vi "Medidor_File3.vi"() -> ()   [LabVIEW 2020]
uses:
  <vilib>/numeric/Random Number (Range) DBL.vi
panel:
  out "Potência C":dbl[](array[numeric])
  out "Corrente C":dbl[](array[numeric])
  out "Tensão C":dbl[](array[numeric])
  out "Potência Ativa C":dbl[](graph)
  out "Potência B":dbl[](array[numeric])
  out "Corrente B":dbl[](array[numeric])
  out "Tensão B":dbl[](array[numeric])
  out "Potência Ativa B":dbl[](graph)
  out "Potência Ativa":dbl[](array[numeric])
  out "Corrente A":dbl[](array[numeric])
  out "Tensão A":dbl[](array[numeric])
  out "Fator de potência":dbl
  in  "Limite inferior fp":dbl
  in  "Limite Superior FP":dbl=100.0
  out "Potência Ativa A":dbl[](graph)
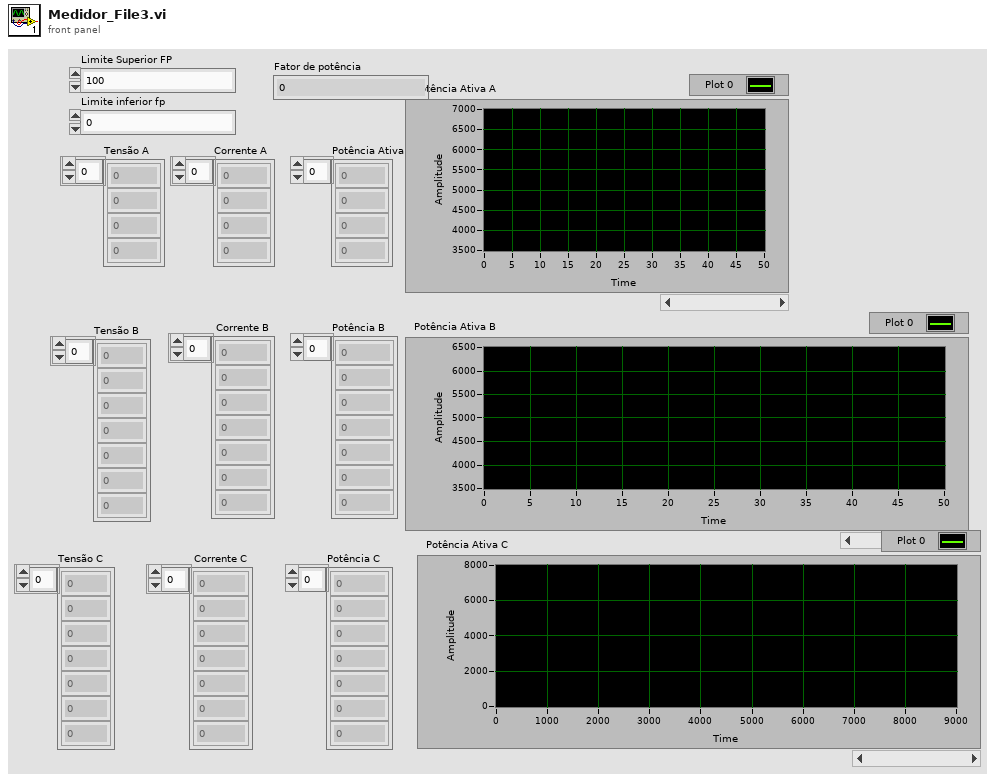
[diagram p1: front panel]
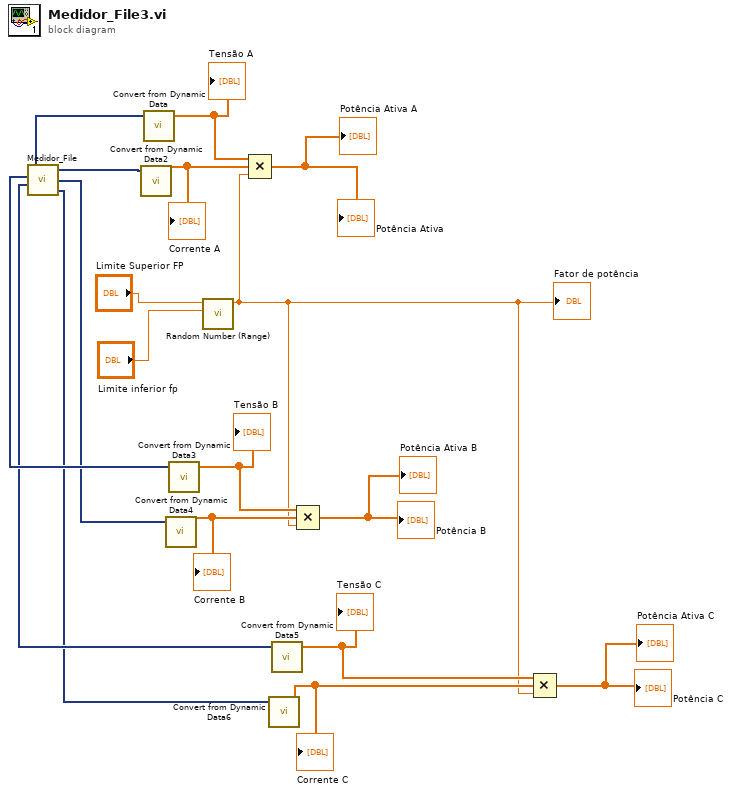
[diagram p0: block diagram]
diagram:
  n1 = call "Medidor_File.vi"() -> ("Corrente Fase C"=w1:dynamicdata, "Corrente Fase B"=w7:dynamicdata, "Corrente Fase A"=w18:dynamicdata, "Tensão Fase C"=w2:dynamicdata, "Tensão Fase B"=w8:dynamicdata, "Tensão Fase A"=w16:dynamicdata)  [unwired: 1 out]
  n2 = call "Convert from Dynamic Data2"("Dynamic Data Type"=w18) -> ("Array"=w17:dbl[])  [unwired: 3 in]
  "Corrente A" <- w17
  n3 = call "Convert from Dynamic Data"("Dynamic Data Type"=w16) -> ("Array"=w15:dbl[])  [unwired: 3 in]
  "Tensão A" <- w15
  n4 = call "Convert from Dynamic Data4"("Dynamic Data Type"=w7) -> ("Array"=w11:dbl[])  [unwired: 3 in]
  "Corrente B" <- w11
  n5 = call "Convert from Dynamic Data3"("Dynamic Data Type"=w8) -> ("Array"=w10:dbl[])  [unwired: 3 in]
  "Tensão B" <- w10
  n6 = call-poly <vilib>:"Random Number (Range).vi"("lower bound (0)"="Limite inferior fp", "upper bound (100)"="Limite Superior FP") -> ("number"=w3:dbl)  [unwired: 9 in]
  "Fator de potência" <- w3
  n7 = Compound Arithmetic op=MULTIPLY(w15, w17, w3) -> (→"Potência Ativa A" →"Potência Ativa":dbl[])
  n8 = call "Convert from Dynamic Data6"("Dynamic Data Type"=w1) -> ("Array"=w6:dbl[])  [unwired: 3 in]
  "Corrente C" <- w6
  n9 = call "Convert from Dynamic Data5"("Dynamic Data Type"=w2) -> ("Array"=w5:dbl[])  [unwired: 3 in]
  "Tensão C" <- w5
  n10 = Compound Arithmetic op=MULTIPLY(w10, w11, w3) -> (→"Potência Ativa B" →"Potência B":dbl[])
  n11 = Compound Arithmetic op=MULTIPLY(w5, w6, w3) -> (→"Potência Ativa C" →"Potência C":dbl[])
